vi "oa_Analog Tacho Hysteresis(1 Channel) with IC.vi"(0 "input signal":dbl[](array[numeric]), 1 "reset? (T)":bool=TRUE, 5 "threshold (auto)":dbl=inf format="%.2f", 7 "slope (Rising)":u16(ring) items=["Rising", "Falling"], 9 "hysteresis(0)":dbl format="%.2f", 11 "initial condition":dbl) -> (4 "output signal":dbl[](array[numeric]), 15 "final condition":dbl)   [LabVIEW 2017, in "SoundVib_TachProcess.lvlib"]
doc: "This VI works like a hysteresis comparater. It can transform the input tachometer signal into a standard square waveform, ignoring small pulsed caused by harmonics or noise. By setting the hystersis value properly, it can make the speed tracking more accurately."
uses:
  <vilib>/addons/Sound and Vibration/Order Analysis/Tach Process/SoundVib_TachProcess.lvlib
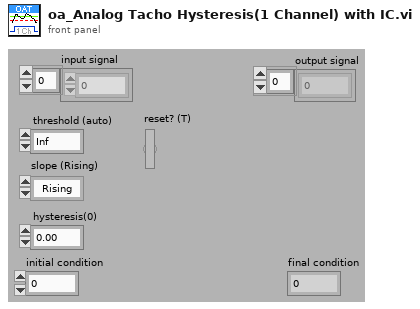
[diagram p1: front panel]
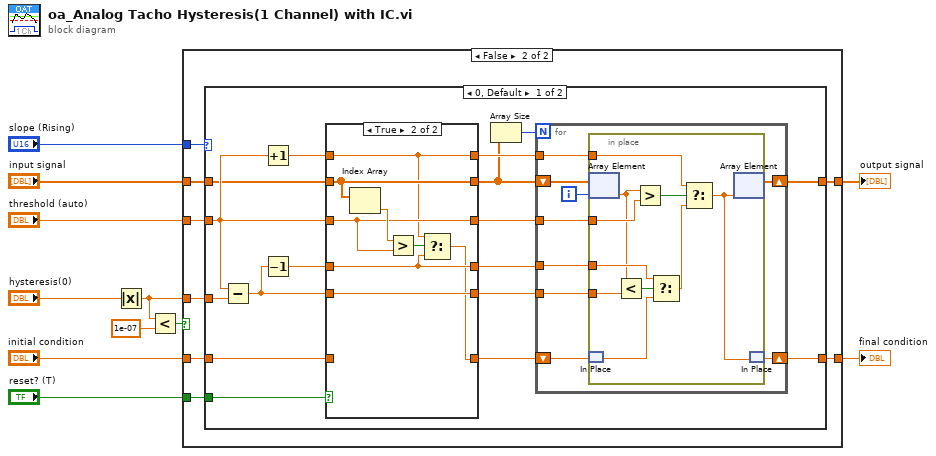
[diagram p0: block diagram]
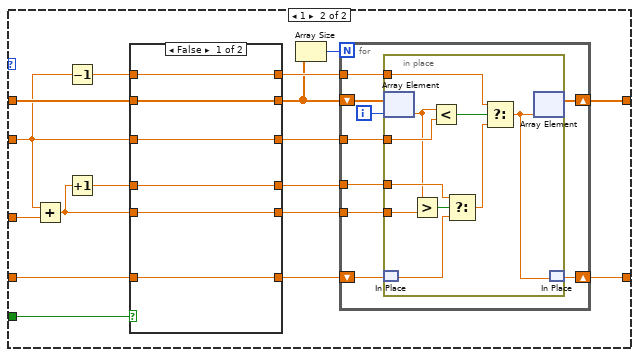
[diagram p4: hidden frame]
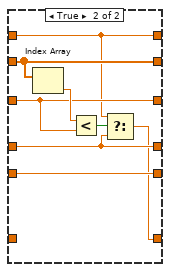
[diagram p5: hidden frame]
diagram:
  n1 = Absolute Value(x="hysteresis(0)") -> (abs(x)=w4:dbl)
  n2 = Less?(x=w4, y=1e-07) -> (x < y?=w6:bool)
  n3 = case shown="False" w6 {
    tunnel: "input signal" -> [w13 w18]
    tunnel: [w13 w17] -> w7
    tunnel: w4 -> [_ w16]
    tunnel: "slope (Rising)" -> [_ w21]
    tunnel: "threshold (auto)" -> [_ w20]
    tunnel: "reset? (T)" -> [_ w19]
    tunnel: "initial condition" -> [w12 w15]
    tunnel: [w12 w14] -> w1
    frame True {
    }
    frame False {
      n4 = case shown="0, Default" w21 {
        tunnel: w18 -> [w33 w88]
        tunnel: w20 -> [w35 w85]
        tunnel: w16 -> [w38 w86]
        tunnel: w19 -> [w32 w81]
        tunnel: [w31 w82] -> w17
        tunnel: w15 -> [w30 w80]
        tunnel: [w29 w79] -> w14
        frame 0, Default {
          n5 = Subtract(x=w35, y=w38) -> (x-y=w36:dbl)
          n6 = Increment(x=w35) -> (x+1=w34:dbl)
          n7 = Decrement(x=w36) -> (x-1=w37:dbl)
          n8 = case shown="True" w32 {
            tunnel: w36 -> [w43 w52]
            tunnel: [w43 w52] -> w28
            tunnel: w37 -> [w42 w46]
            tunnel: [w42 w46] -> w27
            tunnel: w35 -> [w41 w49]
            tunnel: [w41 w49] -> w26
            tunnel: w33 -> [w40 w51]
            tunnel: [w40 w51] -> w23
            tunnel: w34 -> [w39 w47]
            tunnel: [w39 w47] -> w25
            tunnel: w30 -> [w44 _]
            tunnel: [w44 w45] -> w24
            frame False {
            }
            frame True {
              n9 = Index Array(array=w51) -> (element=w50:dbl)  [unwired: 1 in]
              n10 = Greater?(x=w50, y=w49) -> (0:w48:bool)
              n11 = Select(t=w47, s=w48, f=w46) -> (s? t:f=w45:dbl)
            }
          }
          n12 = Array Size(array=w23) -> (size(s)=w22:i32)
          n13 = for {
            N: w22 -> [_]
            tunnel: w26 -> [w61]
            shift-right: [w56] -> w29
            shift-left: w24 -> [w57]
            tunnel: w28 -> [w60]
            tunnel: w25 -> [w59]
            tunnel: w27 -> [w58]
            shift-right: [w53] -> w31
            shift-left: w23 -> [w55]
            i -> [w54]
            n14 = in-place {
              in-place-border: w61 -> [w71]
              in-place-border: w60 -> [w68]
              in-place-border: w59 -> [w67]
              in-place-border: w58 -> [w65]
              n15 = in-place-array #1(w55, w54) -> (w62:dbl)
              n16 = in-place-match #2(w57) -> (w64:dbl)
              n17 = Less?(x=w62, y=w68) -> (x < y?=w69:bool)
              n18 = Greater?(x=w62, y=w71) -> (0:w70:bool)
              n19 = Select(t=w65, s=w69, f=w64) -> (s? t:f=w66:dbl)
              n20 = Select(t=w67, s=w70, f=w66) -> (s? t:f=w63:dbl)
              n21 = in-place-array #1(w63) -> (w53:dbl[])  [unwired: 1 out]
              n22 = in-place-match #2(w63) -> (w56:dbl)
            }
          }
        }
        frame 1 {
          n23 = Add(x=w85, y=w86) -> (x+y=w83:dbl)
          n24 = Decrement(x=w85) -> (x-1=w87:dbl)
          n25 = Increment(x=w83) -> (x+1=w84:dbl)
          n26 = case shown="False" w81 {
            tunnel: w83 -> [w93 w102]
            tunnel: [w93 w102] -> w78
            tunnel: w84 -> [w92 w96]
            tunnel: [w92 w96] -> w77
            tunnel: w85 -> [w91 w99]
            tunnel: [w91 w99] -> w76
            tunnel: w88 -> [w90 w101]
            tunnel: [w90 w101] -> w73
            tunnel: w87 -> [w89 w97]
            tunnel: [w89 w97] -> w75
            tunnel: w80 -> [w94 _]
            tunnel: [w94 w95] -> w74
            frame False {
            }
            frame True {
              n27 = Index Array(array=w101) -> (element=w100:dbl)  [unwired: 1 in]
              n28 = Less?(x=w100, y=w99) -> (x < y?=w98:bool)
              n29 = Select(t=w97, s=w98, f=w96) -> (s? t:f=w95:dbl)
            }
          }
          n30 = Array Size(array=w73) -> (size(s)=w72:i32)
          n31 = for {
            N: w72 -> [_]
            tunnel: w76 -> [w111]
            shift-right: [w106] -> w79
            shift-left: w74 -> [w107]
            tunnel: w78 -> [w110]
            tunnel: w75 -> [w109]
            tunnel: w77 -> [w108]
            shift-right: [w103] -> w82
            shift-left: w73 -> [w105]
            i -> [w104]
            n32 = in-place {
              in-place-border: w111 -> [w121]
              in-place-border: w110 -> [w118]
              in-place-border: w109 -> [w117]
              in-place-border: w108 -> [w115]
              n33 = in-place-array #3(w105, w104) -> (w113:dbl)
              n34 = in-place-match #4(w107) -> (w114:dbl)
              n35 = Greater?(x=w113, y=w118) -> (0:w119:bool)
              n36 = Less?(x=w113, y=w121) -> (x < y?=w120:bool)
              n37 = Select(t=w115, s=w119, f=w114) -> (s? t:f=w116:dbl)
              n38 = Select(t=w117, s=w120, f=w116) -> (s? t:f=w112:dbl)
              n39 = in-place-array #3(w112) -> (w103:dbl[])  [unwired: 1 out]
              n40 = in-place-match #4(w112) -> (w106:dbl)
            }
          }
        }
      }
    }
  }
  "output signal" <- w7
  "final condition" <- w1
